vi "生成机器码.vi"(8 "error in (no error)":errorcluster caption="错误输入（无错误）") -> (0 "error out":errorcluster caption="错误输出", 3 "机器码":string)   [LabVIEW 2014]
uses:
  MD5 Message Digest (Hexadecimal String)__ogtk.vi
panel:
  out "standard output":string caption="标准输出"
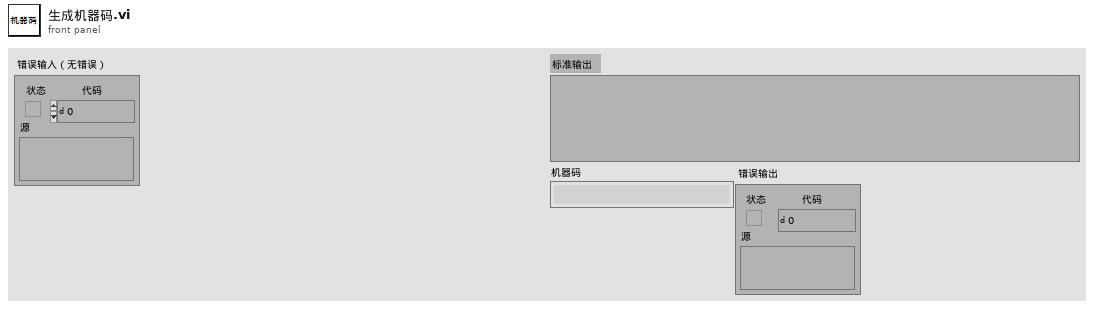
[diagram p1: front panel]
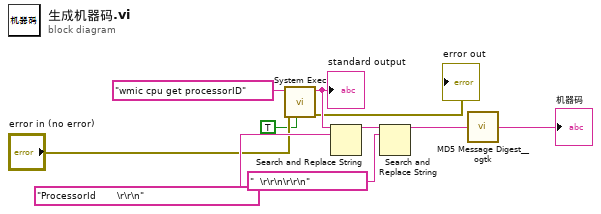
[diagram p0: block diagram]
diagram:
  n1 = call <vilib>:"System Exec.vi"("run minimized? (F)"=TRUE, "error in (no error)"="error in (no error)", "command line"="wmic cpu get processorID") -> ("error out"=→"error out":errorcluster, "standard output"=w9:string)  [unwired: 5 in, 2 out]
  "standard output" <- w9
  n2 = Search and Replace String(input string=w9, search string="ProcessorId       \r\r\n" ("搜索字符串")) -> (result string=w7:string)  [unwired: 6 in, 3 out]
  n3 = Search and Replace String(input string=w7, search string="  \r\r\n\r\r\n" ("搜索字符串")) -> (result string=w5:string)  [unwired: 6 in, 3 out]
  n4 = call-poly "MD5 Message Digest__ogtk.vi"("Message"=w5) -> ("MD5 Message Digest"=→"机器码":string)
